vi "Convert NT String Buffer to LV String.vi"(11 "Buffer":string) -> (3 "String":string)   [LabVIEW 2017]
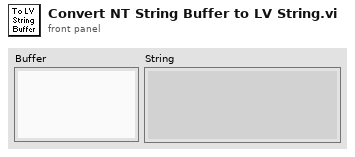
[diagram p1: front panel]
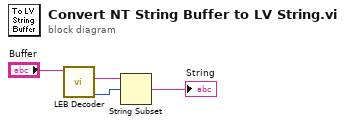
[diagram p0: block diagram]
diagram:
  n1 = call <vilib>:"LEB Decoder.vi"("encoded string"="Buffer") -> ("bytes consumed"=w2:i32, "unmodified string"=w3:string)  [unwired: 8 in, 1 out]
  n2 = String Subset(string=w3, offset (0)=w2) -> (substring=→"String":string)  [unwired: 1 in]
